vi "Initialize.vi"(6 "optional":variant, 8 "error in":errorcluster, 11 "Root in":refnum<class "Root.lvclass">) -> (0 "error out":errorcluster, 3 "Node*":refnum<data-value>)   [LabVIEW 2012, in "Root.lvclass"]
uses:
  Root.lvclass
  <userlib>/XCE/xCE Source/xCE/xceNode/xceNode.lvclass
  <userlib>/XCE/xCE Source/xCE/xceRootNode/xceRootNode.lvclass
  <userlib>/XCE/xCE Source/xCE/xceDataNode/xceDataNode.lvclass
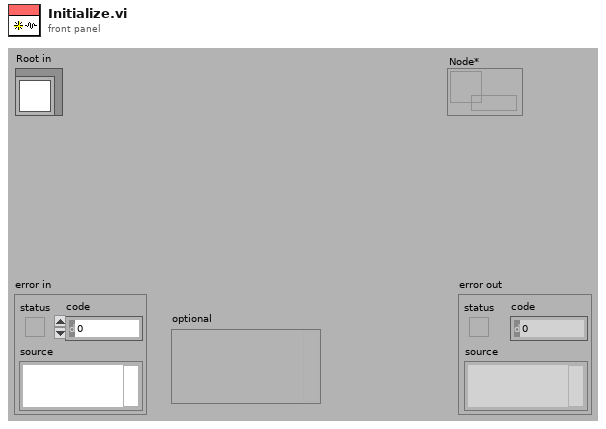
[diagram p1: front panel]
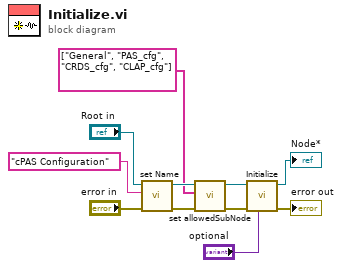
[diagram p0: block diagram]
diagram:
  n1 = call <userlib>:"set Name.vi"("error in (no error)"="error in", "Name"="cPAS Configuration", "xceDataNode in"="Root in") -> ("error out"=w7:errorcluster, "xceDataNode out"=w8:refnum<class "Root.lvclass">)  [unwired: 7 in]
  n2 = call <userlib>:"set allowedSubNode.vi"("error in (no error)"=w7, "Allowed subNode[]"=string[] ["General", "PAS_cfg", "CRDS_cfg", "CLAP_cfg"], "xceDataNode in"=w8) -> ("error out"=w2:errorcluster, "xceDataNode out"=w1:refnum<class "Root.lvclass">)  [unwired: 7 in]
  n3 = call-parent "Initialize.vi"("optional"="optional", "error in"=w2, "xceRootNode in"=w1) -> ("error out"=→"error out":errorcluster, "Node*"=→"Node*":refnum<data-value>)  [unwired: 7 in]
